vi "RT status FPGA Monitoring 2.vi"(8 "error in (no error)":errorcluster, 11 "FPGA VI Reference Out 2":refnum<k20>) -> ()   [LabVIEW 2015]
uses:
  RT/RT Global References.vi
  <vilib>/Utility/error.llb/Error Cluster From Error Code.vi
  <vilib>/rvi/errors/niLvFpgaAdjustHostInterfaceError.vi
  <vilib>/rvi/interface/nirviReadWriteControl/nirviReadWriteControl.xnode
  <vilib>/NI_Real-Time Target Support.lvlib
  <vilib>/Utility/Variable/NI_VariableUtilities.lvlib
  NiFpgaLv.dll
  <vilib>/rvi/interface/Simulation/niFpgaSimulationCallBeginRW.vi
types:
  T1 = typedef "NI_Real-Time Target Support.lvlib/RT CPU Load.ctl" = cluster{"Total (%)":dbl, "Time Critical (%)":dbl, "Timed Structures (%)":dbl, "High (%)":dbl, "Above Normal (%)":dbl, "Normal (%)":dbl, "Background (%)":dbl, "Idle (%)":dbl, "ISR (%)":dbl}
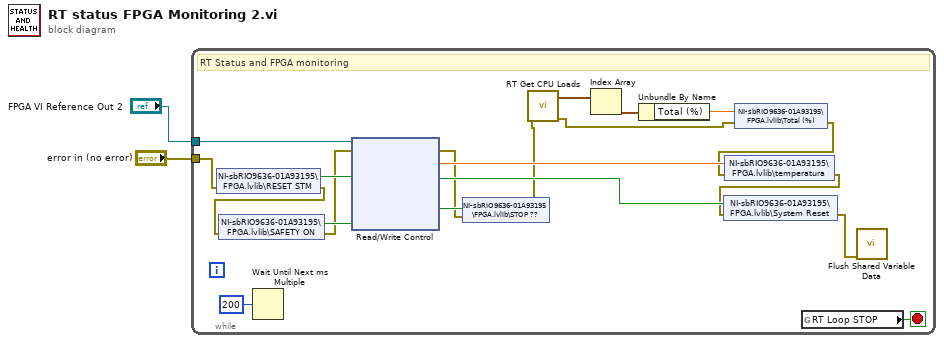
[diagram p0: block diagram]
diagram:
  n1 = while {
    tunnel: "FPGA VI Reference Out 2" -> [w21]
    tunnel: "error in (no error)" -> [w9]
    stop <- w22 stop-if-true
    # "RT Status and FPGA monitoring"
    n2 = shared-variable "NI-sbRIO9636-01A93195\\FPGA.lvlib\\RESET STM"(error in=w9) -> (w11:bool, error out=w4:errorcluster)
    n3 = shared-variable "NI-sbRIO9636-01A93195\\FPGA.lvlib\\SAFETY ON"(error in=w4) -> (w5:bool, error out=w3:errorcluster)
    n4 = Wait Until Next ms Multiple(millisecond multiple=u32 200 ("milliseconds to wait")) -> ()  [unwired: 1 out]
    n5 = xnode "Read/Write Control"("FPGA VI Reference In"=w21, "error in"=w3, "RESET STM"=w11, "SAFETY ON"=w5) -> ("error out"=w7:errorcluster, "temperatura"=w17:sgl, "System Reset"=w13:bool, "STOP ??"=w8:bool)  [unwired: 1 out]
    n6 = shared-variable "NI-sbRIO9636-01A93195\\FPGA.lvlib\\STOP ??"(w8, error in=w7) -> (error out=w6:errorcluster)
    n7 = call <vilib>:"RT Get CPU Loads.vi"("error in (no error)"=w6) -> ("error out"=w16:errorcluster, "CPU loads"=w20:T1[])  [unwired: 9 in]
    n8 = Index Array(array=w20) -> (element=w19:T1)  [unwired: 1 in]
    n9 = Unbundle By Name(w19) -> ("Total (%)"=w18:dbl)
    n10 = shared-variable "NI-sbRIO9636-01A93195\\FPGA.lvlib\\Total (%)"(w18, error in=w16) -> (error out=w15:errorcluster)
    n11 = shared-variable "NI-sbRIO9636-01A93195\\FPGA.lvlib\\temperatura"(w17, error in=w15) -> (error out=w12:errorcluster)
    n12 = shared-variable "NI-sbRIO9636-01A93195\\FPGA.lvlib\\System Reset"(w13, error in=w12) -> (error out=w10:errorcluster)
    n13 = global read "RT Global References.vi" "RT Loop STOP"() -> (w22:bool)
    n14 = call <vilib>:"Flush Shared Variable Data.vi"("error in (no error)"=w10) -> ()  [unwired: 10 in, 1 out]
  }
